vi "Init Device.vi"(8 "error in (no error)":errorcluster, 11 "Orca-Flash 4.0 in":refnum<class "Hamamatsu Camera.lvclass">) -> (0 "error out":errorcluster, 3 "Orca-Flash 4.0 out":refnum<class "Hamamatsu Camera.lvclass">)   [LabVIEW 2018, in "Hamamatsu Camera.lvlib" / "Hamamatsu Camera.lvclass"]
uses:
  Hamamatsu Camera.lvclass
  C:/FlashGordon/Development/Hardware/Camera/Camera.lvclass
  Resources/Type Defs/Physical Camera Assignment.ctl
  Resources/Type Defs/Camera Type.ctl
  Hamamatsu Camera.lvclass/Hamamatsu Camera.ctl
  Resources/GLOBAL/GLOBAL Time-critical.vi
  Camera/Camera.lvclass
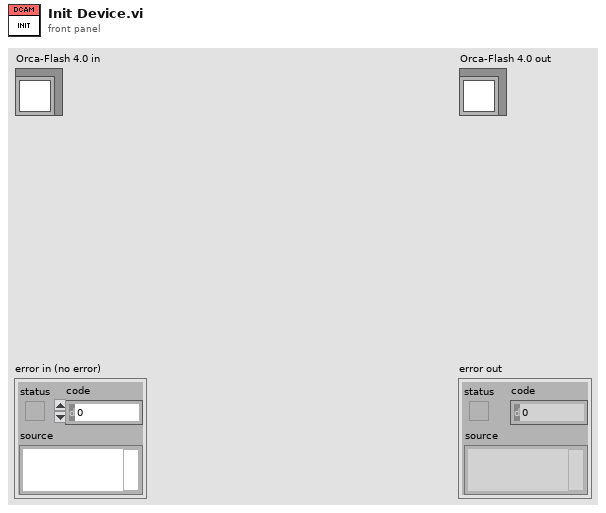
[diagram p1: front panel]
types:
  T1 = typedef "Physical Camera Assignment.ctl" = cluster{"Channel Name":string, "Camera Type":T2, "Serial Number":string, "Flip Vertically":bool, "Flip Horizontally":bool, "photonsPerCount":dbl, "wavelength":i16}
  T2 = typedef "Camera Type.ctl" = enum16{"Hamamatsu"}
  T3 = cluster{"Model":string, "Camera ID":string, "Firmware":string}[]
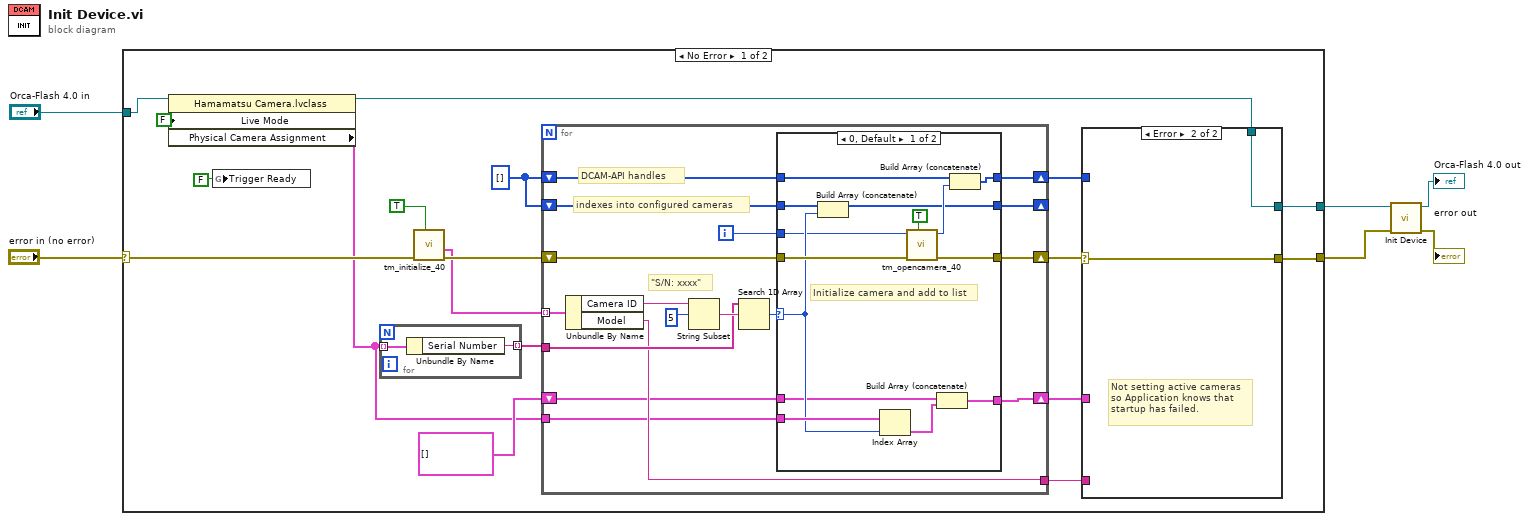
[diagram p0: block diagram]
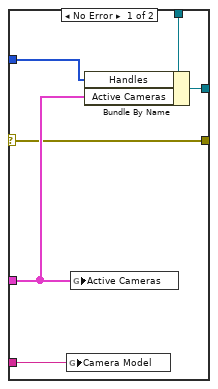
[diagram p2: hidden frame]
diagram:
  n1 = case shown="No Error" "error in (no error)" {
    selector: "error in (no error)" -> [w24 w71]
    tunnel: [w7 w71] -> w1
    tunnel: "Orca-Flash 4.0 in" -> [w17 w70]
    tunnel: [w23 w70] -> w2
    frame No Error {
      w20 = u32[] []
      n2 = property class="Hamamatsu Camera.lvclass"(reference=w17, "Live Mode"=FALSE) -> (reference out=w16:refnum<class "Hamamatsu Camera.lvclass">, "Physical Camera Assignment"=w12:T1[])  [unwired: 1 in, 1 out]
      n3 = global write "GLOBAL Time-critical.vi" "Trigger Ready"(FALSE) -> ()
      n4 = for {
        tunnel: w12 -> [w69] mode=indexing
        tunnel: [w68] -> w22 mode=indexing
        n5 = Unbundle By Name(w69) -> ("Serial Number"=w68:string)
      }
      n6 = call <userlib>:"tm_initialize_40.vi"("HVCC Log (F)"=TRUE, "error in (no error)"=w24) -> ("error out"=w21:errorcluster, "Camera Details Array"=w9:T3)  [unwired: 6 in, 2 out]
      n7 = for {
        tunnel: w9 -> [w49] mode=indexing
        tunnel: w22 -> [w45]
        shift-right: [w42] -> w8
        shift-left: w21 -> [w43]
        shift-right: [w41] -> w18
        shift-left: w20 -> [w38]
        shift-right: [w39] -> _
        shift-left: w20 -> [w40]
        tunnel: [w37] -> w19
        tunnel: w12 -> [w35]
        shift-right: [w36] -> w10
        shift-left: T1[] [] -> [w34]
        i -> [w33]
        # "indexes into configured cameras"
        # "DCAM-API handles"
        # "\"S/N: xxxx\""
        n8 = Unbundle By Name(w49) -> ("Camera ID"=w48:string, "Model"=w37:string)
        n9 = String Subset(string=w48, offset (0)=5) -> (substring=w46:string)  [unwired: 1 in]
        n10 = Search 1D Array(1D array=w45, element=w46) -> (index of element=w44:i32)  [unwired: 1 in]
        n11 = case shown="0, Default" w44 {
          selector: w44 -> [w54 _]
          tunnel: w43 -> [w63 w67]
          tunnel: [w62 w67] -> w42
          tunnel: w38 -> [w58 w66]
          tunnel: [w59 w66] -> w41
          tunnel: w40 -> [w56 w65]
          tunnel: [w55 w65] -> w39
          tunnel: [w53 w64] -> w36
          tunnel: w35 -> [w60 _]
          tunnel: w34 -> [w51 w64]
          tunnel: w33 -> [w50 _]
          frame 0, Default {
            # "Initialize camera and add to list"
            n12 = Build Array (concatenate)(w56, w54) -> (w55:u32[])
            n13 = Index Array(array=w60, index=w54) -> (element=w52:T1)
            n14 = call <userlib>:"tm_opencamera_40.vi"("Force Open"=TRUE, "error in (no error)"=w63, "Camera Index"=w50) -> ("error out"=w62:errorcluster, "Handle out"=w57:u32)  [unwired: 6 in, 1 out]
            n15 = Build Array (concatenate)(w51, w52) -> (w53:T1[])
            n16 = Build Array (concatenate)(w58, w57) -> (w59:u32[])
          }
          frame -1 {
            # "camera not found in config file."
          }
        }
      }
      n17 = case shown="Error" w8 {
        selector: w8 -> [w25 w31]
        tunnel: [w30 w32] -> w23
        tunnel: w19 -> [w29 _]
        tunnel: w18 -> [w28 _]
        tunnel: w16 -> [w27 w32]
        tunnel: w10 -> [w26 _]
        tunnel: [w25 w31] -> w7
        frame No Error {
          n18 = global write "GLOBAL Time-critical.vi" "Camera Model"(w29) -> ()
          n19 = global write "GLOBAL Time-critical.vi" "Active Cameras"(w26) -> ()
          n20 = Bundle By Name(cluster=w27, "Handles"=w28, "Active Cameras"=w26) -> (w30:refnum<class "Hamamatsu Camera.lvclass">)
        }
        frame Error {
          # "Not setting active cameras\nso Application knows that\nstartup has failed."
        }
      }
    }
    frame Error {
    }
  }
  n21 = call-parent "Init Device.vi"("error in (no error)"=w1, "Camera in"=w2) -> ("error out"=→"error out":errorcluster, "Camera out"=→"Orca-Flash 4.0 out":refnum<class "Hamamatsu Camera.lvclass">)  [unwired: 8 in]
